vi "Set Virtual Axis Speed.vi"(7 "Maximum Speed":u32, 8 "error in (no error)":errorcluster, 9 "Device Number":string, 10 "Virtual Axis Number (1)":u8=1, 11 "VISA resource name":refnum<visa-resource-name>) -> (0 "error out":errorcluster, 3 "VISA resource name out":refnum<visa-resource-name>)   [LabVIEW 2013, in "Zaber A Series.lvlib"]
doc: "Sets the maximum speed of a virtual axis that was previously created using the Create Virtual Axis VI. The speed is specified in native device speed units - use the Convert Velocity Units to Device Units VI to convert from standard units.\n\nThis VI requires that the Initialize VI has been called with the same serial port and that the specified virtual axis exists."
uses:
  Zaber A Series.lvlib
  Private/All Commands.ctl
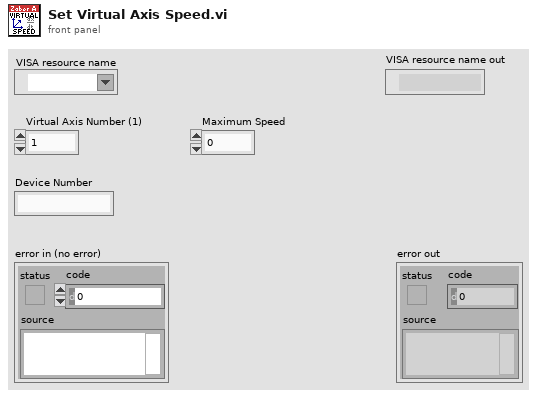
[diagram p1: front panel]
types:
  T1 = typedef "Zaber A Series.lvlib/All Commands.ctl" = string
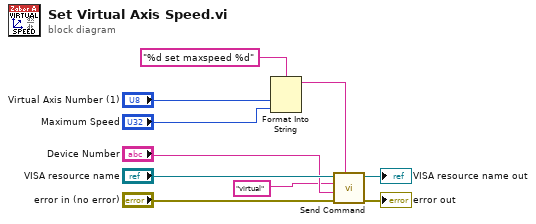
[diagram p0: block diagram]
diagram:
  n1 = Format Into String(format string="%d set maxspeed %d", "Virtual Axis Number (1)", "Maximum Speed") -> (resulting string=w2:string)  [unwired: 2 in, 1 out]
  n2 = call "Send Command.vi"("Data"=w2, "error in (no error)"="error in (no error)", "Device and Axis"="Device Number", "Command"=T1 "virtual" ("Complete Command List"), "VISA resource name"="VISA resource name") -> ("error out"=→"error out":errorcluster, "VISA resource name out"=→"VISA resource name out":refnum<visa-resource-name>)  [unwired: 1 in, 4 out]
